vi "Set Aperture Length.vi"(0 "VISA resource name":refnum<visa-resource-name>, 5 "Aperture Length (s)":dbl=0.1 format="%#.6f", 11 "error in (no error)":errorcluster) -> (4 "VISA resource name out":refnum<visa-resource-name>, 15 "error out":errorcluster)   [LabVIEW 2020, in "NH Research Regenerative Test Series.lvlib"]
doc: "Specifies how long a measurement aperture is desired to be in seconds. A measurement aperture is the total length of the capture. The Module will pick the sample rate. The actual number of samples may be less than that specified in Set Max Samples.vi. Applies to both voltage and current measurements."
uses:
  NH Research Regenerative Test Series.lvlib
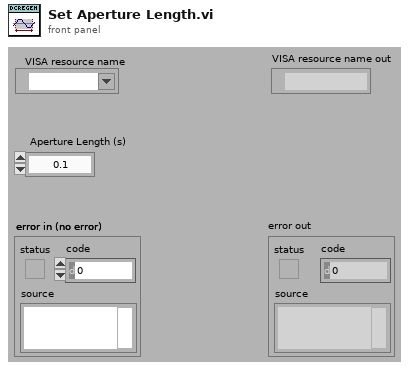
[diagram p1: front panel]
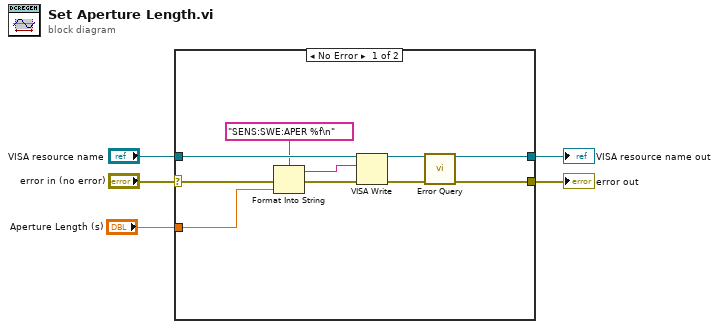
[diagram p0: block diagram]
diagram:
  n1 = case shown="No Error" "error in (no error)" {
    selector: "error in (no error)" -> [w9 w17]
    tunnel: "VISA resource name" -> [w15 w16]
    tunnel: [w14 w16] -> w4
    tunnel: [w13 w17] -> w3
    tunnel: "Aperture Length (s)" -> [w7 _]
    frame No Error {
      n2 = Format Into String(format string="SENS:SWE:APER %f\n" ("Command"), error in=w9, w7) -> (resulting string=w6:string, error out=w8:errorcluster)  [unwired: 1 in]
      n3 = VISA Write(VISA resource name=w15, write buffer=w6, error in (no error)=w8) -> (VISA resource name out=w12:refnum<visa-resource-name>, error out=w11:errorcluster)  [unwired: 1 out]
      n4 = call "Error Query.vi"("VISA resource name"=w12, "error in (no error)"=w11) -> ("VISA resource name out"=w14:refnum<visa-resource-name>, "error out"=w13:errorcluster)  [unwired: 10 in, 2 out]
    }
    frame Error {
    }
  }
  "error out" <- w3
  "VISA resource name out" <- w4
